vi "Stability.vi"(4 "Array":dbl[](array[numeric]) format="%.6p") -> (1 "Stability":dbl format="%.6p")   [LabVIEW 2019]
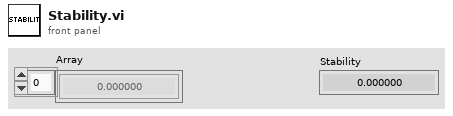
[diagram p1: front panel]
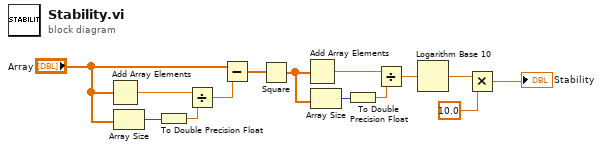
[diagram p0: block diagram]
diagram:
  n1 = Add Array Elements(numeric array="Array") -> (sum=w14:dbl)
  n2 = Array Size(array="Array") -> (size(s)=w13:i32)
  n3 = To Double Precision Float(number=w13) -> (double precision float=w12:dbl)
  n4 = Divide(x=w14, y=w12) -> (x/y=w10:dbl)
  n5 = Subtract(x="Array", y=w10) -> (x-y=w9:dbl[])
  n6 = Square(x=w9) -> (x^2=w5:dbl[])
  n7 = Add Array Elements(numeric array=w5) -> (sum=w6:dbl)
  n8 = Array Size(array=w5) -> (size(s)=w7:i32)
  n9 = To Double Precision Float(number=w7) -> (double precision float=w8:dbl)
  n10 = Divide(x=w6, y=w8) -> (x/y=w4:dbl)
  n11 = Logarithm Base 10(1:w4) -> (0:w3:dbl)
  n12 = Multiply(x=w3, y=10.0) -> (x*y=→"Stability":dbl)
